vi "Load Plugin Dialog.vi"(6 "Plugin Selection Ring Text":string, 7 "Window Title":string, 8 "error in (no error)":errorcluster, 10 "Plugin List":T1[](array[typedef])=[{"Plugin Name"="", "Controller Type"=enum."Invalid", "Control Panel Path"=path "", "Plugin Type"=enum."Optimizer"}, {"Plugin Name"="", "Controller Type"=enum."Invalid", "Control Panel Path"=path "", "Plugin Type"=enum."Optimizer"}, {"Plugin Name"="", "Controller Type"=enum."Invalid", "Control Panel Path"=path "", "Plugin Type"=enum."Optimizer"}], 11 "Plugin Selection Ring":u16(ring) caption="Select Hardware" items=["ChromTech MX-Class", "ChromTech Series I", "ChromTech Series III", "Mock Pump Controller", "Mock Temperature Controller", "Omega Platinum Series", "Polar Bear", "Mock Pump Controller", "Abort VI Test Pump Controller", "Mock Pump Controller (from source plugins/)"]) -> (0 "error out":errorcluster, 1 "cancelled":bool, 2 "Instance Name":string, 3 "Plugin Selected":T1={"Plugin Name"="", "Controller Type"=enum."Invalid", "Control Panel Path"=path "", "Plugin Type"=enum."Optimizer"})   [LabVIEW 2020]
doc: "Dialog allowing the user to select a plugin by name. Returns the selected plugin details."
uses:
  Plugin Manager/Plugin Details.ctl
  Controller/Controller Type.ctl
  Plugin Manager/Plugin Types.ctl
  Plugin Manager/Plugin Manager.lvlib
  Controller/Generic Plugin.lvclass
panel:
  in  "Plugin Label (blank for default)":string
  in  "Cancel Btn":bool
  in  "OK Btn":bool
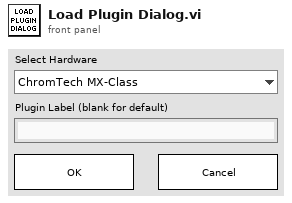
[diagram p1: front panel]
types:
  T1 = typedef "Plugin Manager.lvlib/Plugin Details.ctl" = cluster{"Plugin Name":string, "Controller Type":T2, "Control Panel Path":path, "Plugin Type":T3}
  T2 = typedef "Generic Plugin.lvclass/Controller Type.ctl" = enum16{"Invalid", "Temperature Controller", "Pump Controller", "Generic Optimizer", "LC Parser"}
  T3 = typedef "Plugin Manager.lvlib/Plugin Types.ctl" = enum16{"Invalid", "Optimizer", "Analyzer", "Hardware"}
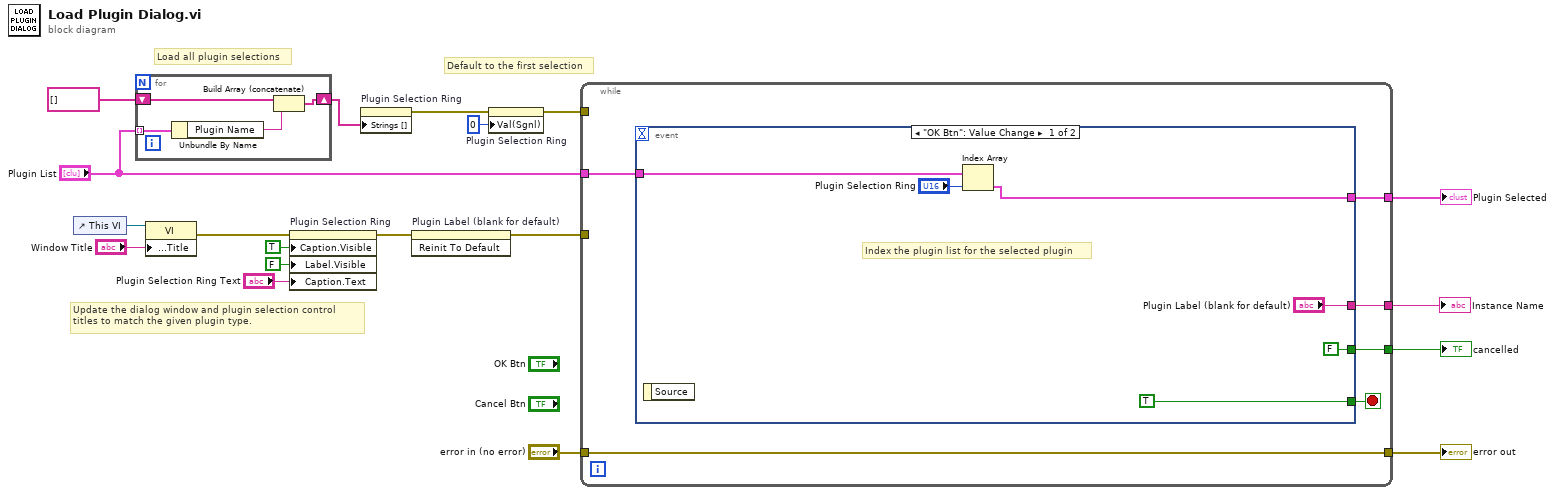
[diagram p0: block diagram]
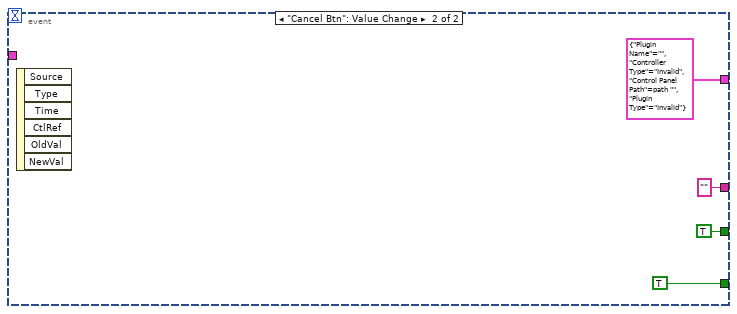
[diagram p2: hidden frame]
diagram:
  # "Update the dialog window and plugin selection control\ntitles to match the given plugin type."
  # "Default to the first selection"
  # "Load all plugin selections"
  n1 = control-ref of="This VI"() -> (w8:refnum<vi>)
  n2 = for {
    tunnel: "Plugin List" -> [w23] mode=indexing
    shift-right: [w20] -> w13
    shift-left: string[] [] -> [w21]
    n3 = Unbundle By Name(w23) -> ("Plugin Name"=w22:string)
    n4 = Build Array (concatenate)(w21, w22) -> (w20:string[])
  }
  n5 = property class="VI"(reference=w8, "Front Panel.Title"="Window Title") -> (error out=w9:errorcluster)  [unwired: 1 in, 1 out]
  n6 = property on="Plugin Selection Ring" class="Ring (strict)"(error in=w9, "Caption.Visible"=TRUE, "Label.Visible"=FALSE, "Caption.Text"="Plugin Selection Ring Text") -> (error out=w2:errorcluster)  [unwired: 1 in, 1 out]
  n7 = property on="Plugin Selection Ring" class="Ring (strict)"("Strings []"=w13) -> (error out=w19:errorcluster)  [unwired: 2 in, 1 out]
  n8 = invoke on="Plugin Label (blank for default)" class="Str" method="Reinit To Default"(error in=w2) -> (error out=w1:errorcluster)  [unwired: 2 in, 2 out]
  n9 = property on="Plugin Selection Ring" class="Ring (strict)"(error in=w19, "Val(Sgnl)"=u16 0 ("Value (Signaling)")) -> (error out=w18:errorcluster)  [unwired: 1 in, 1 out]
  n10 = while {
    tunnel: [w28] -> w10
    tunnel: w18 -> [_]
    tunnel: "Plugin List" -> [w27]
    tunnel: [w26] -> w16
    tunnel: "error in (no error)" -> [w26]
    tunnel: [w25] -> w11
    tunnel: [w24] -> w3
    tunnel: w1 -> [_]
    stop <- w29 stop-if-true
    n11 = event shown="[0] \"OK Btn\": Value Change" {
      selector: _ -> [_ _]
      dyn-events: _ -> [_ _]
      timeout: _ -> [_ _]
      tunnel: [TRUE TRUE] -> w29
      tunnel: [w33 T1 {"Plugin Name"="", "Controller Type"=enum."Invalid", "Control Panel Path"=path "", "Plugin Type"=enum."Invalid"}] -> w28
      tunnel: w27 -> [w34 _]
      tunnel: [FALSE TRUE] -> w25
      tunnel: ["Plugin Label (blank for default)" "" ("Plugin Label (blank for default)")] -> w24
      event "OK Btn": Value Change {
        # "Index the plugin list for the selected plugin"
        n12 = event-data() -> ()  [unwired: 1 in, 1 out]
        n13 = Index Array(array=w34, index="Plugin Selection Ring") -> (element=w33:T1)
      }
      event "Cancel Btn": Value Change {
        n14 = event-data() -> ()  [unwired: 1 in, 6 out]
      }
    }
  }
  "error out" <- w16
  "cancelled" <- w11
  "Plugin Selected" <- w10
  "Instance Name" <- w3
